vi "Engine - Read Properties.vi"(8 "error in (no error)":errorcluster, 10 "DMM-Switch Configuration In":T1={"DMM Resource Name"="", "DMM Measurement"=enum."DC Volts", "DMM Resolution in Digits"=6.5, "DMM Range [EU]"=10.0, "Switch Resource Name"="", "Switch Topology"="2503/2-Wire 24x1 Mux", "Switch Scan List"="ab0->com0 & com0->ch0:2;", "Switch Trigger Source"=enum."TTL0", "Switch Scan Advanced Output"=enum."TTL1", "DMM Measurement Complete"=enum."TTL 0", "DMM Trigger Source"=enum."TTL 1", "# of Channels"=0, "Group CH Names - Configuration"="", "Group CH Names - Input Channels"="", "Group CH Names - Measurement Channels"="", "Group CH Names - Runtime Status"=""} {"DMM Resolution in Digits" items=["3 1/2"=3.5, "4 1/2"=4.5, "5 1/2"=5.5, "6 1/2"=6.5, "7 1/2"=7.5]}, 11 "Specified Channel Ref List In":T9[](array[typedef]) format="%.0x") -> (0 "error out":errorcluster, 2 "DMM-Switch Configuration Out":T1 {"DMM Resolution in Digits" items=["3 1/2"=3.5, "4 1/2"=4.5, "5 1/2"=5.5, "6 1/2"=6.5, "7 1/2"=7.5]}, 3 "Specified Channel Ref List Out":T9[](array[typedef]) format="%.0x")   [LabVIEW 2015, in "DMM-SWITCH-ScanList Engine.lvlib"]
doc: "Reads all properties from Input Configuration Channels (DMM, Switch, and Triggering) and writes them into the DMM-Switch Configuration Cluster"
uses:
  DMM-SWITCH-ScanList Engine.lvlib
  TypeDefs/DMM-Switch Configuration.ctl
  <instrlib>/niDMM/nidmm.llb/niDMM Function.ctl
  <instrlib>/niDMM/nidmm.llb/niDMM Resolution in Digits.ctl
  <instrlib>/niSwitch/niSwitch.LLB/niSwitch Topologies.ctl
  <instrlib>/niSwitch/niSwitch.LLB/niSwitch Trigger Input.ctl
  <instrlib>/niSwitch/niSwitch.LLB/niSwitch Scan Advanced Output.ctl
  <instrlib>/niDMM/nidmm.llb/niDMM Measurement Complete.ctl
  <instrlib>/niDMM/nidmm.llb/niDMM Trigger.ctl
  <vilib>/NI Veristand/Custom Device API/Custom Device Item Ref.ctl
  Shared/Constants.vi
  <vilib>/NI Veristand/Custom Device API/Get Item Property (String).vi
  <vilib>/NI Veristand/Custom Device API/Get Item Property (String Array).vi
  <vilib>/NI Veristand/Custom Device API/Get Item Property (U16).vi
  <vilib>/NI Veristand/Custom Device API/Get Item Property (Double).vi
  <vilib>/NI Veristand/Custom Device API/Custom Device API.lvlib
  Shared/DMM-SWITCH-ScanList Shared.lvlib
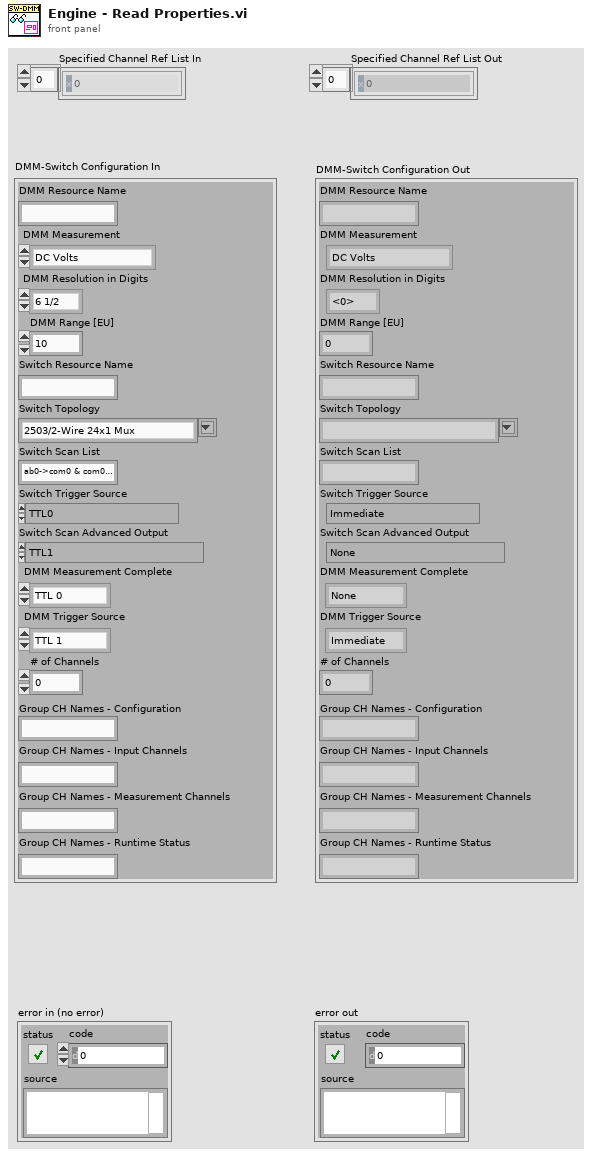
[diagram p1: front panel]
types:
  T1 = typedef "DMM-SWITCH-ScanList Engine.lvlib/DMM-Switch Configuration.ctl" = cluster{"DMM Resource Name":string, "DMM Measurement":T2, "DMM Resolution in Digits":T3, "DMM Range [EU]":dbl, "Switch Resource Name":string, "Switch Topology":T4, "Switch Scan List":string, "Switch Trigger Source":T5, "Switch Scan Advanced Output":T6, "DMM Measurement Complete":T7, "DMM Trigger Source":T8, "# of Channels":u32, "Group CH Names - Configuration":string, "Group CH Names - Input Channels":string, "Group CH Names - Measurement Channels":string, "Group CH Names - Runtime Status":string}
  T2 = typedef "niDMM Function.ctl" = enum16{"DC Volts", "AC Volts", "DC Current", "AC Current", "2-wire Resistance", "4-wire Resistance", "Diode", "Frequency", "Period", "AC Volts DC Coupled", "Capacitance", "Inductance", "Temperature"}
  T3 = typedef "niDMM Resolution in Digits.ctl" = dbl
  T4 = typedef "niSwitch Topologies.ctl" = string
  T5 = typedef "niSwitch Trigger Input.ctl" = enum16{"Immediate", "External", "TTL0", "TTL1", "TTL2", "TTL3", "TTL4", "TTL5", "TTL6", "TTL7", "ECL0", "ECL1", "PXI Star", "Software Trigger Function", "Rear Connector", "Front Connector", "Rear Connector of Module 1", "Rear Connector of Module 2", "Rear Connector of Module 3", "Rear Connector of Module 4", "Rear Connector of Module 5", "Rear Connector of Module 6", "Rear Connector of Module 7", "Rear Connector of Module 8", "Rear Connector of Module 9", "Rear Connector of Module 10", "Rear Connector of Module 11", "Rear Connector of Module 12", "Front Connector of Module 1", "Front Connector of Module 2", "Front Connector of Module 3", "Front Connector of Module 4", "Front Connector of Module 5", "Front Connector of Module 6", "Front Connector of Module 7", "Front Connector of Module 8", "Front Connector of Module 9", "Front Connector of Module 10", "Front Connector of Module 11", "Front Connector of Module 12"}
  T6 = typedef "niSwitch Scan Advanced Output.ctl" = enum16{"None", "External", "TTL0", "TTL1", "TTL2", "TTL3", "TTL4", "TTL5", "TTL6", "TTL7", "ECL0", "ECL1", "PXI Star", "Rear Connector", "Front Connector", "Rear Connector Module 1", "Rear Connector Module 2", "Rear Connector Module 3", "Rear Connector Module 4", "Rear Connector Module 5", "Rear Connector Module 6", "Rear Connector Module 7", "Rear Connector Module 8", "Rear Connector Module 9", "Rear Connector Module 10", "Rear Connector Module 11", "Rear Connector Module 12", "Front Connector Module 1", "Front Connector Module 2", "Front Connector Module 3", "Front Connector Module 4", "Front Connector Module 5", "Front Connector Module 6", "Front Connector Module 7", "Front Connector Module 8", "Front Connector Module 9", "Front Connector Module 10", "Front Connector Module 11", "Front Connector Module 12"}
  T7 = typedef "niDMM Measurement Complete.ctl" = enum16{"None", "External", "TTL 0", "TTL 1", "TTL 2", "TTL 3", "TTL 4", "TTL 5", "TTL 6", "TTL 7", "LBR Trig 0"}
  T8 = typedef "niDMM Trigger.ctl" = enum16{"Immediate", "External", "TTL 0", "TTL 1", "TTL 2", "TTL 3", "TTL 4", "TTL 5", "TTL 6", "Software", "TTL 7", "PXI Star", "LBR Trig 1", "Aux Trig 1"}
  T9 = typedef "Custom Device API.lvlib/Custom Device Item Ref.ctl" = u64
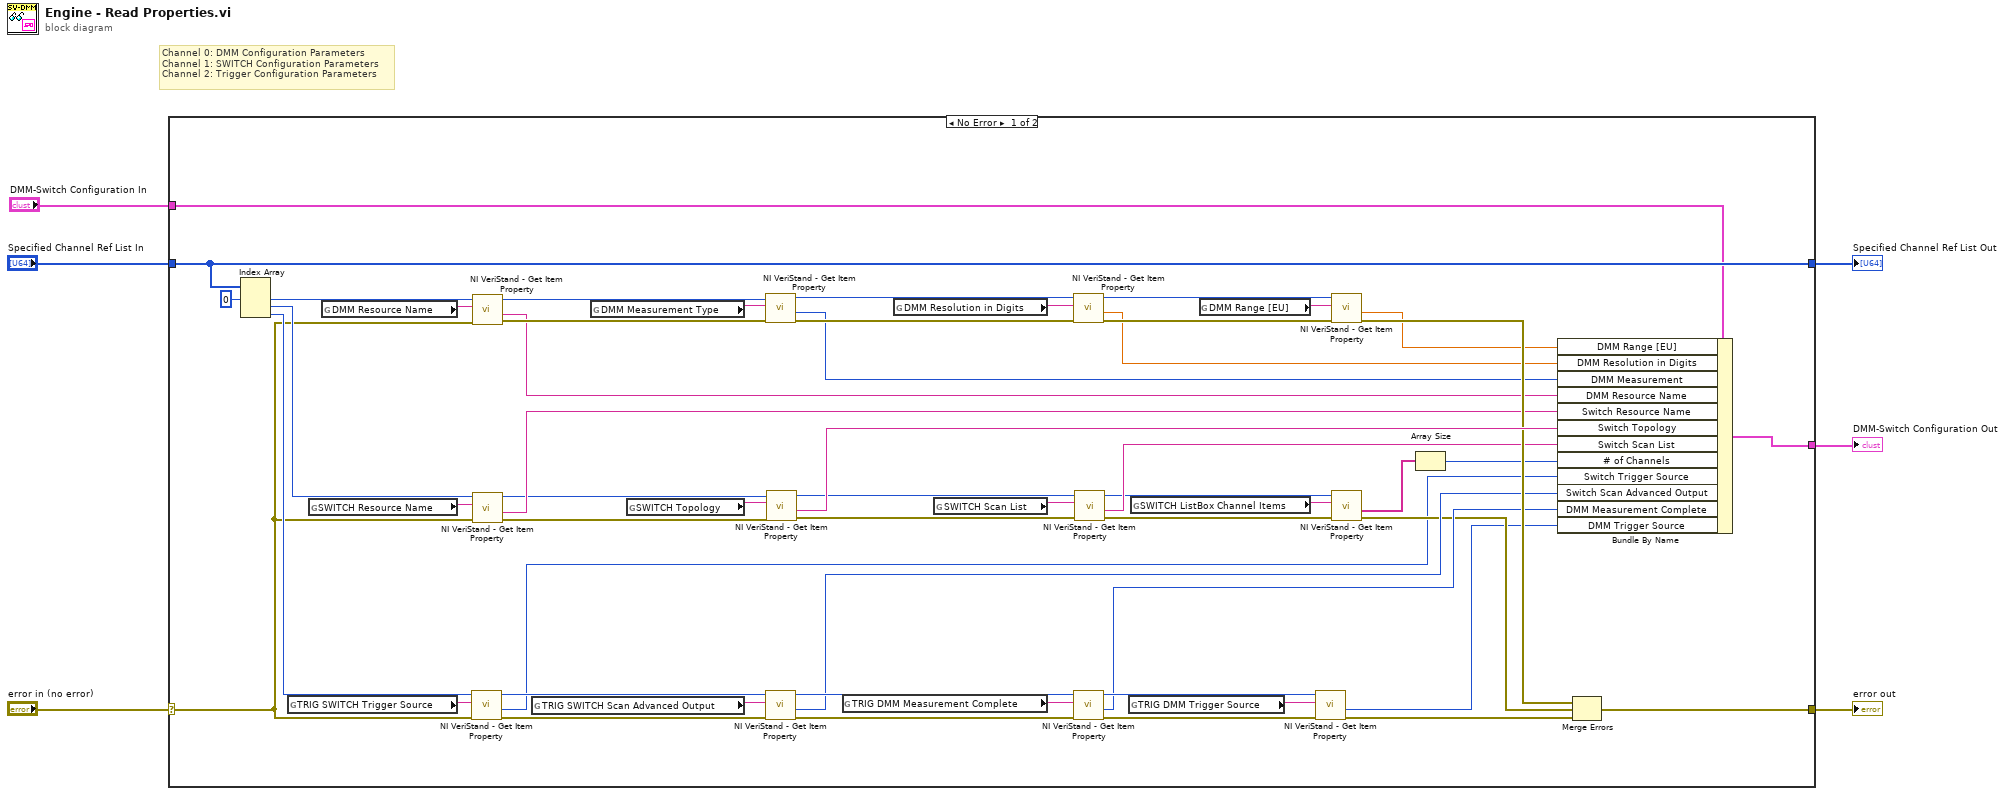
[diagram p0: block diagram]
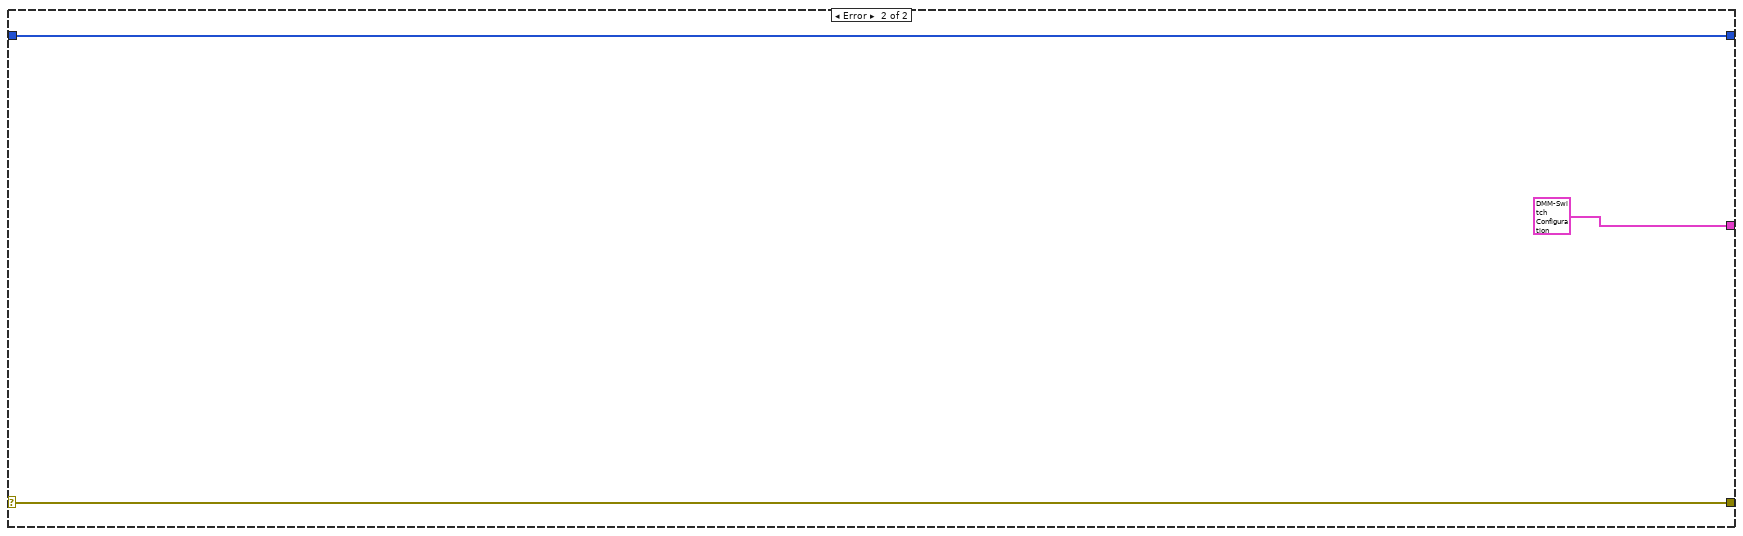
[diagram p2: hidden frame]
diagram:
  # "Channel 0: DMM Configuration Parameters\nChannel 1: SWITCH Configuration Parameters\nChannel 2: Trigger Configuration Parameters"
  n1 = case shown="No Error" "error in (no error)" {
    selector: "error in (no error)" -> [w33 w64]
    tunnel: [w60 w64] -> w6
    tunnel: [w58 T1 {"DMM Resource Name"="", "DMM Measurement"=enum."DC Volts", "DMM Resolution in Digits"=6.5, "DMM Range [EU]"=10.0, "Switch Resource Name"="", "Switch Topology"="2503/2-Wire 24x1 Mux", "Switch Scan List"="ab0->com0 & com0->ch0:2;", "Switch Trigger Source"=enum."TTL0", "Switch Scan Advanced Output"=enum."TTL1", "DMM Measurement Complete"=enum."TTL 0", "DMM Trigger Source"=enum."TTL 1", "# of Channels"=0, "Group CH Names - Configuration"="", "Group CH Names - Input Channels"="", "Group CH Names - Measurement Channels"="", "Group CH Names - Runtime Status"=""} ("DMM-Switch Configuration")] -> w5
    tunnel: "Specified Channel Ref List In" -> [w32 w63]
    tunnel: [w32 w63] -> w2
    tunnel: "DMM-Switch Configuration In" -> [w8 _]
    frame No Error {
      n2 = Index Array(array=w32, index #1=0 ("index")) -> (element #1=w41:T9, element #2=w49:T9, element #3=w50:T9)  [unwired: 2 in]
      n3 = global read "Constants.vi" "TRIG SWITCH Trigger Source"() -> (w22:string)
      n4 = global read "Constants.vi" "SWITCH Resource Name"() -> (w23:string)
      n5 = global read "Constants.vi" "DMM Resource Name"() -> (w24:string)
      n6 = call-poly <vilib>:"NI VeriStand - Get Item Property.vi"("error in (no error)"=w33, "Property Name"=w22, "Item Ref in"=w50) -> ("error out"=w47:errorcluster, "Value"=w28:u16, "Item Ref out"=w55:T9)  [unwired: 5 in, 1 out]
      n7 = call-poly <vilib>:"NI VeriStand - Get Item Property.vi"("error in (no error)"=w33, "Property Name"=w24, "Item Ref in"=w41) -> ("error out"=w40:errorcluster, "Value"=w10:string, "Item Ref out"=w39:T9)  [unwired: 5 in, 1 out]
      n8 = call-poly <vilib>:"NI VeriStand - Get Item Property.vi"("error in (no error)"=w33, "Property Name"=w23, "Item Ref in"=w49) -> ("error out"=w45:errorcluster, "Value"=w51:string, "Item Ref out"=w44:T9)  [unwired: 5 in, 1 out]
      n9 = global read "Constants.vi" "TRIG SWITCH Scan Advanced Output"() -> (w19:string)
      n10 = global read "Constants.vi" "DMM Measurement Type"() -> (w21:string)
      n11 = global read "Constants.vi" "SWITCH Topology"() -> (w20:string)
      n12 = call-poly <vilib>:"NI VeriStand - Get Item Property.vi"("error in (no error)"=w40, "Property Name"=w21, "Item Ref in"=w39) -> ("error out"=w37:errorcluster, "Value"=w11:u16, "Item Ref out"=w38:T9)  [unwired: 5 in, 1 out]
      n13 = call-poly <vilib>:"NI VeriStand - Get Item Property.vi"("error in (no error)"=w47, "Property Name"=w19, "Item Ref in"=w55) -> ("error out"=w48:errorcluster, "Value"=w53:u16, "Item Ref out"=w56:T9)  [unwired: 5 in, 1 out]
      n14 = call-poly <vilib>:"NI VeriStand - Get Item Property.vi"("error in (no error)"=w45, "Property Name"=w20, "Item Ref in"=w44) -> ("error out"=w42:errorcluster, "Value"=w61:string, "Item Ref out"=w43:T9)  [unwired: 5 in, 1 out]
      n15 = global read "Constants.vi" "TRIG DMM Measurement Complete"() -> (w18:string)
      n16 = global read "Constants.vi" "DMM Resolution in Digits"() -> (w16:string)
      n17 = global read "Constants.vi" "SWITCH Scan List"() -> (w17:string)
      n18 = call-poly <vilib>:"NI VeriStand - Get Item Property.vi"("error in (no error)"=w37, "Property Name"=w16, "Item Ref in"=w38) -> ("error out"=w35:errorcluster, "Value"=w12:dbl, "Item Ref out"=w36:T9)  [unwired: 5 in, 1 out]
      n19 = call-poly <vilib>:"NI VeriStand - Get Item Property.vi"("error in (no error)"=w48, "Property Name"=w18, "Item Ref in"=w56) -> ("error out"=w46:errorcluster, "Value"=w54:u16, "Item Ref out"=w57:T9)  [unwired: 5 in, 1 out]
      n20 = call-poly <vilib>:"NI VeriStand - Get Item Property.vi"("error in (no error)"=w42, "Property Name"=w17, "Item Ref in"=w43) -> ("error out"=w31:errorcluster, "Value"=w52:string, "Item Ref out"=w29:T9)  [unwired: 5 in, 1 out]
      n21 = global read "Constants.vi" "TRIG DMM Trigger Source"() -> (w9:string)
      n22 = global read "Constants.vi" "SWITCH ListBox Channel Items"() -> (w14:string)
      n23 = global read "Constants.vi" "DMM Range [EU]"() -> (w15:string)
      n24 = call-poly <vilib>:"NI VeriStand - Get Item Property.vi"("error in (no error)"=w46, "Property Name"=w9, "Item Ref in"=w57) -> ("error out"=w7:errorcluster, "Value"=w25:u16)  [unwired: 5 in, 2 out]
      n25 = call-poly <vilib>:"NI VeriStand - Get Item Property.vi"("error in (no error)"=w35, "Property Name"=w15, "Item Ref in"=w36) -> ("error out"=w59:errorcluster, "Value"=w13:dbl)  [unwired: 5 in, 2 out]
      n26 = call-poly <vilib>:"NI VeriStand - Get Item Property.vi"("error in (no error)"=w31, "Property Name"=w14, "Item Ref in"=w29) -> ("error out"=w30:errorcluster, "Value"=w27:string[])  [unwired: 5 in, 2 out]
      n27 = Array Size(array=w27) -> (size(s)=w26:i32)
      n28 = Bundle By Name(cluster=w8, "DMM Range [EU]"=w13, "DMM Resolution in Digits"=w12, "DMM Measurement"=w11, "DMM Resource Name"=w10, "Switch Resource Name"=w51, "Switch Topology"=w61, "Switch Scan List"=w52, "# of Channels"=w26, "Switch Trigger Source"=w28, "Switch Scan Advanced Output"=w53, "DMM Measurement Complete"=w54, "DMM Trigger Source"=w25) -> (w58:T1)
      n29 = Merge Errors(w59, w30, w7) -> (w60:errorcluster)
    }
    frame Error {
    }
  }
  "error out" <- w6
  "DMM-Switch Configuration Out" <- w5
  "Specified Channel Ref List Out" <- w2
